vi "_ RunMe.vi"() -> ()   [LabVIEW 2020]
panel:
  in  "Image":path=path "images/Test BMP Image.bmp"
  in  "Dest Format":string(combo)="{6fddc324-4e03-4bfe-b185-3d77768dc90e}"
  out "Image":T1(plugin-control)
  out "Image Stride":u32
  out "Image Height":u32
  out "Image Width":u32
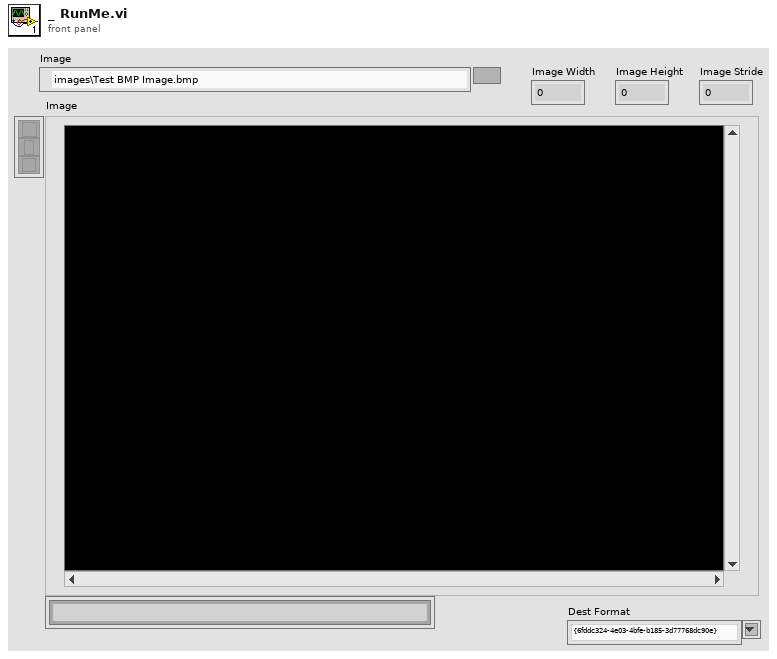
[diagram p1: front panel]
types:
  T1 = typedef "IMAQ Image.ctl" = refnum<image>
  T2 = typedef "Image Type" = u32
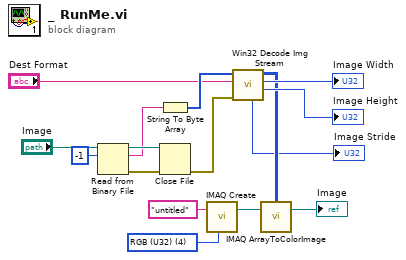
[diagram p0: block diagram]
diagram:
  w8 = T2 4 items=["Grayscale (U8)", "Grayscale (I16)", "Grayscale (SGL)", "Complex (CSG)", "RGB (U32)", "HSL (U32)", "RGB (U64)", "Grayscale (U16)"] ("Image Type")
  n1 = Read from Binary File(10:-1 ("count (1)"), 11:"Image") -> (0:w2:errorcluster, 2:w13:string, 3:w14:refnum<file>)  [unwired: 4 in, 1 out]
  n2 = String To Byte Array(string=w13) -> (unsigned byte array=w12:u8[])
  n3 = Close File(refnum=w14, error in=w2) -> (error out=w1:errorcluster)  [unwired: 1 out]
  n4 = call "IMAQ Create"("Image Name"="untitled", "Image Type"=w8) -> ("New Image"=w7:T1)  [unwired: 3 in, 1 out]
  n5 = call "Win32 Decode Img Stream.vi"("error in (no error)"=w1, "Dest Format"="Dest Format", "Image Data"=w12) -> ("Image Height"=→"Image Height":u32, "Image Width"=→"Image Width":u32, "Dest"=w5:u32[][], "Image Stride"=→"Image Stride":u32)  [unwired: 4 in, 1 out]
  n6 = call "IMAQ ArrayToColorImage"("Image Pixels (U32)"=w5, "Image"=w7) -> ("Image Out"=→"Image":T1)  [unwired: 3 in, 1 out]
